vi "image_processing.vi"() -> ()   [LabVIEW 2018]
uses:
  <vilib>/picture/picture.llb/imagedata.ctl
  <vilib>/Analysis/2dsp.llb/2D Convolution (DBL).vi
  <vilib>/picture/picture.llb/Draw 8-Bit Pixmap.vi
  <vilib>/Analysis/NI_AALPro.lvlib
panel:
  out "new picture 3":picture
  out "new picture 2":picture
  out "new picture":picture
  out "image data":T1
  in  "Path":path=path "C:/Users/HMK/Desktop/tp_matlab/TP_Labview/Image_Processing/cameraman.png"
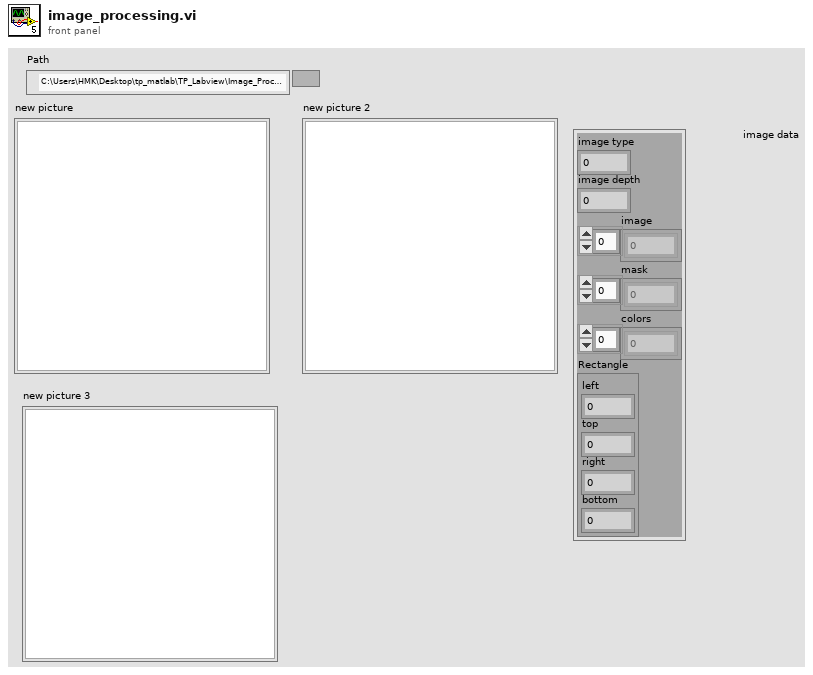
[diagram p1: front panel]
types:
  T1 = typedef "imagedata.ctl" = cluster{"image type":i32, "image depth":i32, "image":u8[], "mask":u8[], "colors":u32[], "Rectangle":cluster{"left":i16, "top":i16, "right":i16, "bottom":i16}}
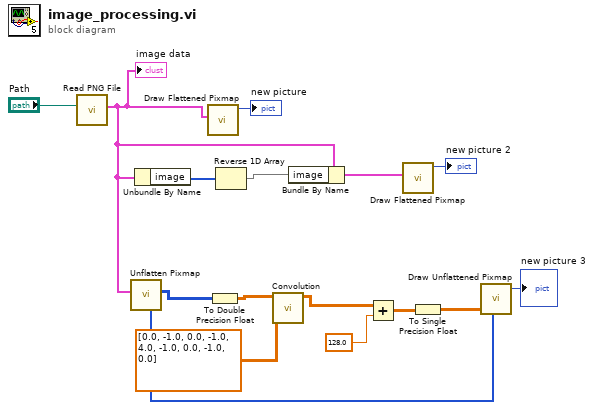
[diagram p0: block diagram]
diagram:
  n1 = call <vilib>:"Read PNG File.vi"("path to PNG file"="Path") -> ("image data"=w10:T1)  [unwired: 8 in, 2 out]
  "image data" <- w10
  n2 = call <vilib>:"Unflatten Pixmap.vi"("image data"=w10) -> ("8-bit pixmap"=w9:u8[][], "colors"=w1:u32[])  [unwired: 4 in, 5 out]
  n3 = Unbundle By Name(w10) -> ("image"=w14:u8[])
  n4 = call <vilib>:"Draw Flattened Pixmap.vi"("image data"=w10) -> ("new picture"=→"new picture":picture)  [unwired: 8 in]
  n5 = To Double Precision Float(number=w9) -> (double precision float=w8:dbl[][])
  n6 = Reverse 1D Array(array=w14) -> (reversed array=w13:u8[])
  n7 = call-poly <vilib>:"Convolution.vi"("Y"=dbl[][] [[0.0, -1.0, 0.0], [-1.0, 4.0, -1.0], [0.0, -1.0, 0.0]], "X"=w8) -> ("X * Y"=w5:dbl[][])  [unwired: 8 in, 1 out]
  n8 = Bundle By Name(cluster=w10, "image"=w13) -> (w11:T1)
  n9 = Add(x=w5, y=128.0) -> (x+y=w4:dbl[][])
  n10 = call <vilib>:"Draw Flattened Pixmap.vi"("image data"=w11) -> ("new picture"=→"new picture 2":picture)  [unwired: 8 in]
  n11 = To Single Precision Float(number=w4) -> (single precision float=w3:sgl[][])
  n12 = call-poly <vilib>:"Draw Unflattened Pixmap.vi"("data"=w3, "color table"=w1) -> ("new picture"=→"new picture 3":picture)  [unwired: 7 in]
